vi "Generate Update Thing JSON.vi"(4 "Expected Version":i32, 6 "Merge Attributes":bool, 9 "Type Operation":T1, 10 "Type":string, 11 "Attributes":T2[](array[typedef])) -> (3 "Create Thing JSON":string)   [LabVIEW 2015, in "NI_AWS_IoT.lvlib"]
uses:
  NI_AWS_IoT.lvlib
  Core/HTTP Request/Name Value Pair.ctl
  Type Operation.ctl
  Core/HTTP Request/HTTP Request.lvclass
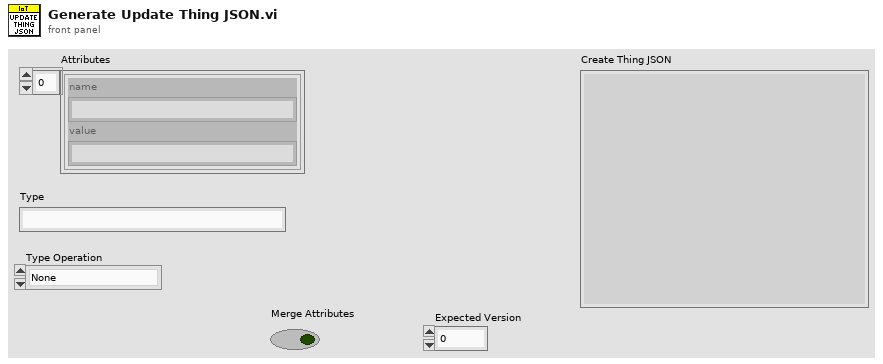
[diagram p1: front panel]
types:
  T1 = typedef "NI_AWS_IoT.lvlib/Type Operation.ctl" = enum16{"None", "Update Type", "Remove Type"}
  T2 = typedef "NI_AWS_Core.lvlib/HTTP Request.lvclass/Name Value Pair.ctl" = cluster{"name":string, "value":string}
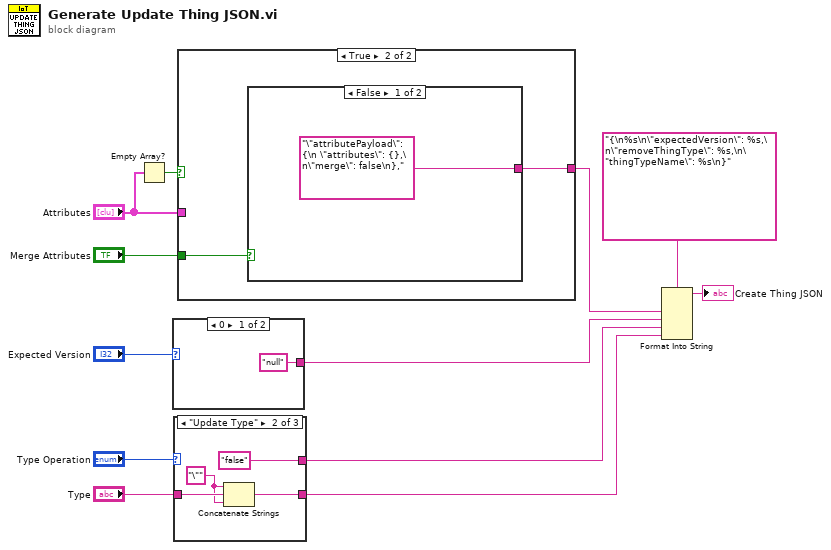
[diagram p0: block diagram]
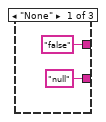
[diagram p2: hidden frame]
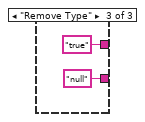
[diagram p3: hidden frame]
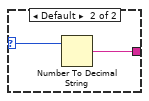
[diagram p4: hidden frame]
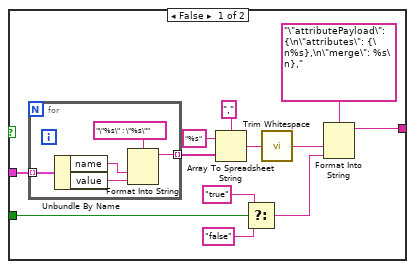
[diagram p5: hidden frame]
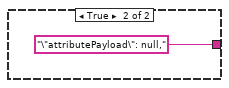
[diagram p6: hidden frame]
diagram:
  n1 = Empty Array?(array="Attributes") -> (empty?=w8:bool)
  n2 = case shown="0" "Expected Version" {
    selector: "Expected Version" -> [_ w15]
    tunnel: ["null" w14] -> w5
    frame 0 {
    }
    frame Default {
      n3 = Number To Decimal String(number=w15) -> (decimal integer string=w14:string)  [unwired: 1 in]
    }
  }
  n4 = case shown="\"Update Type\"" "Type Operation" {
    tunnel: "Type" -> [_ w20 _]
    tunnel: ["false" "false" "true"] -> w2
    tunnel: ["null" ("Type") w19 "null" ("Type")] -> w1
    frame "None" {
    }
    frame "Update Type" {
      w18 = "\""
      n5 = Concatenate Strings(w18, w20, w18) -> (w19:string)
    }
    frame "Remove Type" {
    }
  }
  n6 = case shown="True" w8 {
    tunnel: [w29 w42] -> w10
    tunnel: "Attributes" -> [w28 _]
    tunnel: "Merge Attributes" -> [w27 w41]
    frame False {
      n7 = for {
        tunnel: w28 -> [w40] mode=indexing
        tunnel: [w36] -> w35 mode=indexing
        n8 = Unbundle By Name(w40) -> ("name"=w37:string, "value"=w38:string)
        n9 = Format Into String(format string="\"%s\" : \"%s\"", w37, w38) -> (resulting string=w36:string)  [unwired: 2 in, 1 out]
      }
      n10 = Array To Spreadsheet String(delimiter (Tab)=",", array=w35, 3:"%s" ("format string")) -> (spreadsheet string=w34:string)
      n11 = Select(t="true", s=w27, f="false") -> (s? t:f=w24:string)
      n12 = call <vilib>:"Trim Whitespace.vi"("string"=w34) -> ("trimmed string"=w31:string)  [unwired: 1 in]
      n13 = Format Into String(format string="\"attributePayload\": {\n\"attributes\": {\n%s},\n\"merge\": %s\n},", w31, w24) -> (resulting string=w29:string)  [unwired: 2 in, 1 out]
    }
    frame True {
      n14 = case shown="False" w41 {
        tunnel: ["\"attributePayload\": {\n \"attributes\": {},\n\"merge\": false\n}," "\"attributePayload\": null,"] -> w42
        frame False {
        }
        frame True {
        }
      }
    }
  }
  n15 = Format Into String(format string="{\n%s\n\"expectedVersion\": %s,\n\"removeThingType\": %s,\n\"thingTypeName\": %s\n}", w10, w5, w2, w1) -> (resulting string=→"Create Thing JSON":string)  [unwired: 2 in, 1 out]
